vi "32 GPS Time Code Parser (2017).vi"(1 "GPS Time Code":string, 4 "CPU Time In":dbl format="%#.6f") -> (7 "Latitude":string, 8 "Clock ID":string, 9 "Latitude Sign":string, 10 "GPS Time":string, 11 "Longitude":string, 12 "GPS Date":string, 13 "Longitude Sign":string, 14 "Labview Time":dbl format="%#.3f", 15 "GPS Lock":bool, 16 "CPU Time":dbl format="%#.6f", 17 "PLL Freq":string, 18 "Last Good Lock":string)   [LabVIEW 2017]
panel:
  out "Time Valid (A/V)":string
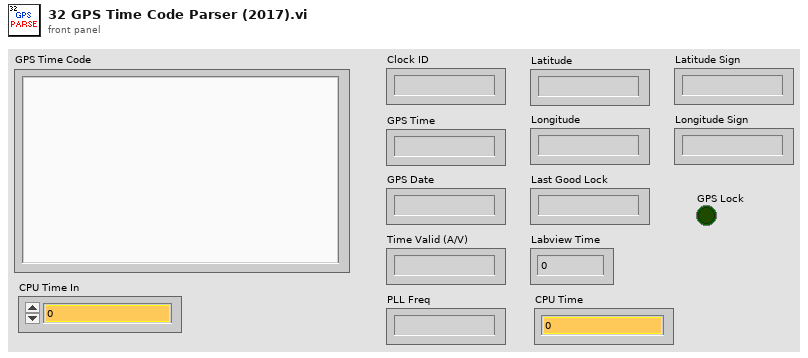
[diagram p1: front panel]
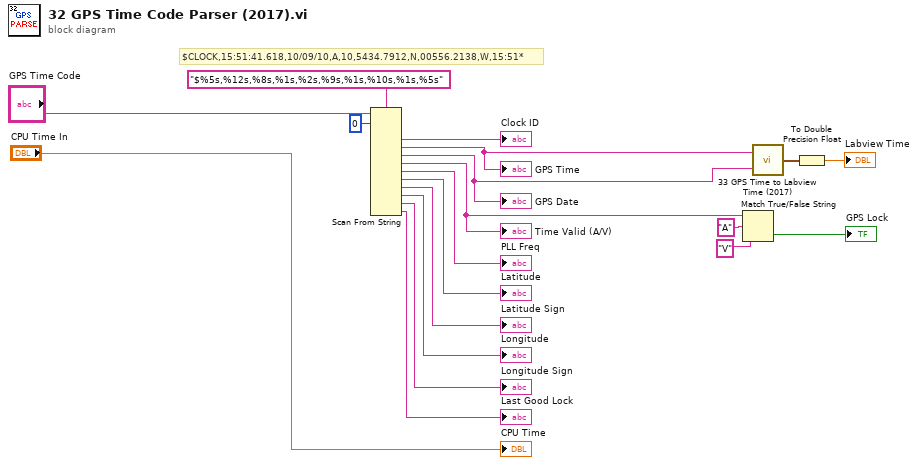
[diagram p0: block diagram]
diagram:
  # "$CLOCK,15:51:41.618,10/09/10,A,10,5434.7912,N,00556.2138,W,15:51*"
  n1 = Scan From String(format string="$%5s,%12s,%8s,%1s,%2s,%9s,%1s,%10s,%1s,%5s", input string="GPS Time Code", initial scan location=u32 0) -> (output 1=→"Clock ID":string, output 2=w3:string, output 3=w2:string, output 4=w6:string, output 5=→"PLL Freq":string, output 6=→"Latitude":string, output 7=→"Latitude Sign":string, output 8=→"Longitude":string, output 9=→"Longitude Sign":string, output 10=→"Last Good Lock":string)  [unwired: 11 in, 3 out]
  "GPS Time" <- w3
  "GPS Date" <- w2
  "Time Valid (A/V)" <- w6
  n2 = Match True/False String(2:"V" ("false string"), 3:"A" ("true string"), 4:w6) -> (0:→"GPS Lock":bool)  [unwired: 1 out]
  n3 = call "33 GPS Time to Labview Time (2017).vi"("GPS Date"=w2, "GPS Time"=w3) -> ("Labview Time Stamp"=w1:timestamp)
  n4 = To Double Precision Float(number=w1) -> (double precision float=→"Labview Time":dbl)
  "CPU Time" <- "CPU Time In"
